vi "callchain.vi"(11 "note":string) -> ()   [LabVIEW 2011]
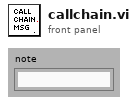
[diagram p1: front panel]
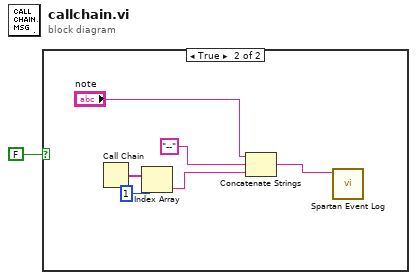
[diagram p0: block diagram]
diagram:
  n1 = case shown="True" FALSE {
    frame False {
    }
    frame True {
      n2 = Call Chain() -> (call chain=w7:string[])
      n3 = Index Array(array=w7, index=1) -> (element=w3:string)
      n4 = Concatenate Strings("note", "--", w3) -> (w6:string)
      n5 = call "Spartan Event Log.vi"("message (\"\")"=w6) -> ()  [unwired: 7 in, 1 out]
    }
  }
